vi "Generate_FP_Snapshot.vi"(6 "TabControl in":refnum<vi>, 7 "directory copy":path, 8 "error in":errorcluster, 11 "Generated File Path":path) -> (0 "error out":errorcluster)   [LabVIEW 2020]
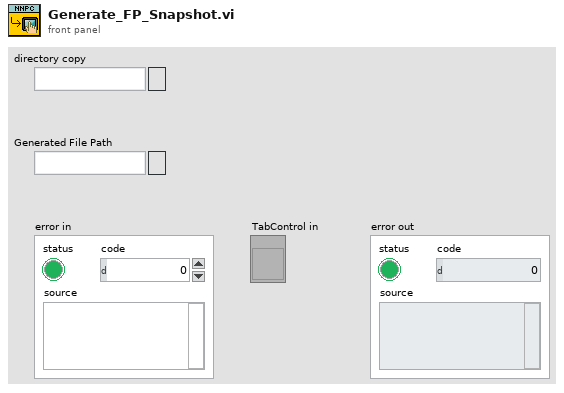
[diagram p1: front panel]
types:
  T1 = typedef "imagedata.ctl" = cluster{"image type":i32, "image depth":i32, "image":u8[], "mask":u8[], "colors":u32[], "Rectangle":cluster{"left":i16, "top":i16, "right":i16, "bottom":i16}}
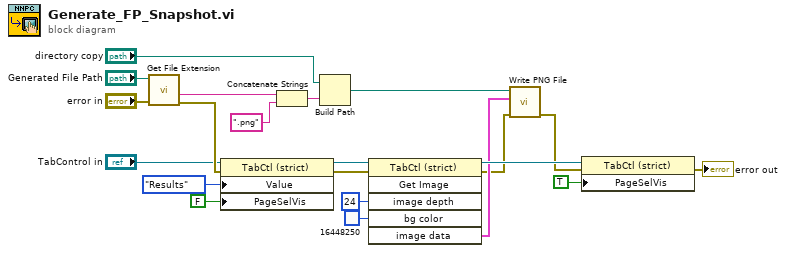
[diagram p0: block diagram]
diagram:
  n1 = call <vilib>:"Get File Extension.vi"("error in (no error)"="error in", "file"="Generated File Path") -> ("error out"=w20:errorcluster, "filename without extension"=w3:string)  [unwired: 5 in, 3 out]
  n2 = property class="TabCtl (strict)"(reference="TabControl in", error in=w20, "Value"=enum32{"Setup", "Results"}."Results", "PageSelVis"=FALSE ("Page Selector Visible")) -> (reference out=w14:refnum<vi>, error out=w15:errorcluster)
  n3 = Concatenate Strings(w3, ".png" ("string")) -> (w5:string)
  n4 = Build Path(base path="directory copy", name or relative path=w5) -> (appended path=w6:path)
  n5 = invoke class="TabCtl (strict)" method="Get Image"(reference=w14, error in=w15, "image depth"=24 ("Image Depth"), "bg color"=u32 16448250 ("Background Color")) -> (reference out=w21:refnum<vi>, error out=w11:errorcluster, "image data"=w12:T1)  [unwired: 2 in, 3 out]
  n6 = call <vilib>:"Write PNG File.vi"("error in (no error)"=w11, "image data"=w12, "path to PNG file"=w6) -> ("error out"=w17:errorcluster)  [unwired: 7 in, 1 out]
  n7 = property class="TabCtl (strict)"(reference=w21, error in=w17, "PageSelVis"=TRUE ("Page Selector Visible")) -> (error out=→"error out":errorcluster)  [unwired: 1 out]
